vi "Subset.vi"(7 "length (-1: rest)":i64=-1 format="%d bytes", 8 "error in (no error)":errorcluster, 9 "offset (0)":u64 format="%d bytes", 10 "subset Pointer type":refnum<class "Pointer.lvclass">, 11 "base Pointer in":refnum<class "Pointer.lvclass">) -> (0 "error out":errorcluster, 1 "offset out":u64 format="%d bytes", 2 "subset Pointer":refnum<class "Pointer.lvclass">, 3 "base Pointer out":refnum<class "Pointer.lvclass">)   [LabVIEW 2020, in "Memory Manager.lvlib" / "Pointer.lvclass"]
doc: "Creates a new <b>subset Pointer</b> object that represents a subset of the provided <b>base Pointer</b> block."
uses:
  Pointer.lvclass
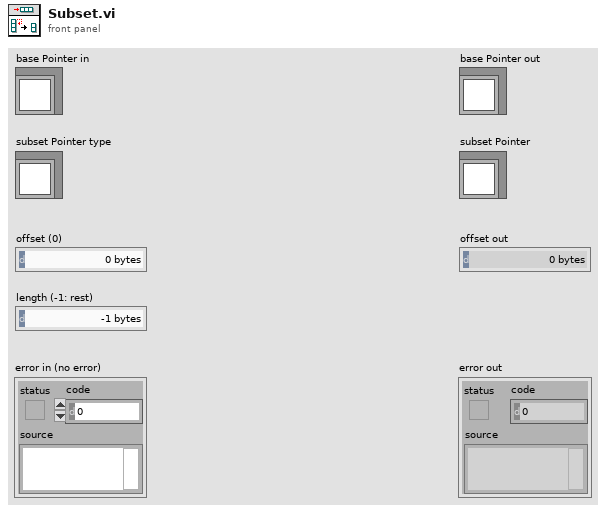
[diagram p1: front panel]
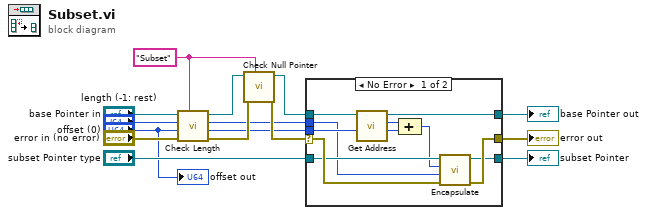
[diagram p0: block diagram]
diagram:
  w3 = "Subset" ("source vi name")
  n1 = call "Check Length.vi"("source vi name"=w3, "error in (no error)"="error in (no error)", "offset (0)"="offset (0)", "length (-1: rest)"="length (-1: rest)", "Pointer in"="base Pointer in") -> ("error out"=w15:errorcluster, "offset"=w6:u64, "size"=w7:u64, "Pointer out"=w5:refnum<class "Pointer.lvclass">)  [unwired: 3 in]
  n2 = call "Check Null Pointer.vi"("source vi name"=w3, "error in (no error)"=w15, "Pointer in"=w5) -> ("error out"=w14:errorcluster, "Pointer out"=w4:refnum<class "Pointer.lvclass">)  [unwired: 7 in]
  n3 = case shown="No Error" w14 {
    selector: w14 -> [w25 w26]
    tunnel: "subset Pointer type" -> [w24 w27]
    tunnel: [w22 w27] -> w9
    tunnel: w4 -> [w21 w28]
    tunnel: [w20 w28] -> w8
    tunnel: w7 -> [w16 _]
    tunnel: w6 -> [w19 _]
    tunnel: [w23 w26] -> w2
    frame No Error {
      n4 = call "Get Address.vi"("Pointer in"=w21) -> ("address"=w18:u64, "Pointer out"=w20:refnum<class "Pointer.lvclass">)  [unwired: 9 in]
      n5 = Compound Arithmetic op=ADD(w18, w19) -> (w17:u64)
      n6 = call "Encapsulate.vi"("error in (no error)"=w25, "size"=w16, "address"=w17, "Pointer type"=w24) -> ("error out"=w23:errorcluster, "Pointer"=w22:refnum<class "Pointer.lvclass">)  [unwired: 6 in]
    }
    frame Error {
    }
  }
  "error out" <- w2
  "subset Pointer" <- w9
  "base Pointer out" <- w8
  "offset out" <- "offset (0)"
